vi "alignment by unt corner.vi"(8 "error in (no error)":errorcluster) -> (0 "error out":errorcluster, 3 "angle Z":ext, 5 "ant corner 2":ext, 11 "ant corner":ext)   [LabVIEW 2017]
uses:
  <vilib>/myRIO/Instrument Drivers/Onboard IO/I2C/typedefs/I2C Reference.ctl
  <vilib>/myRIO/Common/Instrument Driver Framework/Utilities/typedefs/myRIO Generic Hardware Reference.ctl
  <vilib>/myRIO/Common/Instrument Driver Framework/Utilities/typedefs/Hardware Version Enum.ctl
  <vilib>/myRIO/Common/Instrument Driver Framework/Utilities/typedefs/myRIO v1.0 Reference.ctl
  <vilib>/myRIO/Common/Instrument Driver Framework/Utilities/typedefs/Generic FPGA Reference.ctl
  <vilib>/myRIO/Common/Instrument Driver Framework/myRIO v1.0/I2C/typedefs/I2C Channels Enum.ctl
  <vilib>/myRIO/Instrument Drivers/Onboard IO/I2C/typedefs/I2C Configuration.ctl
  <vilib>/myRIO/Instrument Drivers/Onboard IO/I2C/typedefs/I2C Transfer Rate.ctl
  <vilib>/userdefined/High Color/nirio_resource_hc.ctl
  <vilib>/myRIO/Instrument Drivers/Onboard IO/DIO/typedefs/DIO Reference.ctl
  <vilib>/myRIO/Common/Instrument Driver Framework/myRIO v1.0/DIO/typedefs/DIO Channels List.ctl
  <vilib>/myRIO/Common/Instrument Driver Framework/myRIO v1.0/DIO/typedefs/DIO Channels Enum.ctl
  <vilib>/myRIO/Common/Instrument Driver Framework/myRIO v1.0/I2C/vis/myRIO v1.1 Open I2C.vi
  <vilib>/myRIO/Common/Instrument Driver Framework/Utilities/vis/Is FPGA Ref Available.vi
  <vilib>/myRIO/Common/Instrument Driver Framework/myRIO v1.0/DIO/vis/myRIO v1.1 Open DIO.vi
  <vilib>/myRIO/Instrument Drivers/Onboard IO/DIO/vis/Write.vi
  <vilib>/myRIO/Common/Instrument Driver Framework/Utilities/vis/Validate Channels.vi
  <vilib>/myRIO/Common/Instrument Driver Framework/myRIO v1.0/I2C/vis/myRIO v1.0 Reserve I2C.vi
  <vilib>/myRIO/Common/Instrument Driver Framework/myRIO v1.0/DIO/vis/myRIO v1.0 Reserve DIO.vi
  <vilib>/myRIO/Common/Instrument Driver Framework/myRIO v1.0/I2C/vis/myRIO v1.0 Close I2C.vi
  <vilib>/myRIO/Common/Instrument Driver Framework/myRIO v1.0/I2C/vis/myRIO v1.0 Build MUX Configuration I2C.vi
  <vilib>/myRIO/Common/Instrument Driver Framework/myRIO v1.0/Resource Manager/vis/myRIO v1.0 Reserve Channel List.vi
  <vilib>/myRIO/Common/Instrument Driver Framework/myRIO v1.0/DIO/vis/myRIO v1.0 Build MUX Configuration DIO.vi
  <vilib>/myRIO/Common/Instrument Driver Framework/myRIO v1.0/I2C/vis/myRIO v1.0 Unreserve I2C.vi
  <vilib>/myRIO/Common/Instrument Driver Framework/myRIO v1.0/Resource Manager/vis/myRIO v1.0 Create Configuration List.vi
  <vilib>/myRIO/Common/Instrument Driver Framework/myRIO v1.0/Resource Manager/vis/myRIO v1.0 Reserve Channel.vi
  <vilib>/myRIO/Common/Instrument Driver Framework/myRIO v1.0/Resource Manager/vis/myRIO v1.0 Unreserve Channel.vi
  <vilib>/myRIO/Common/Instrument Driver Framework/myRIO v1.0/Resource Manager/vis/myRIO v1.0 Unreserve Channel List.vi
  <vilib>/myRIO/Common/Instrument Driver Framework/myRIO v1.0/Resource Manager/vis/myRIO v1.0 Build Mutex Name.vi
  <vilib>/Utility/VariantDataType/GetNumericInfo.vi
  <vilib>/Utility/error.llb/Error Cluster From Error Code.vi
  <vilib>/myRIO/Common/Instrument Driver Framework/myRIO v1.0/myRIO v1.1 Open.vi
  <vilib>/myRIO/Common/Instrument Driver Framework/Utilities/vis/IO Manager.vi
  <vilib>/myRIO/Common/Instrument Driver Framework/Utilities/vis/Configuration Manager.vi
  <vilib>/myRIO/Common/Instrument Driver Framework/myRIO v1.0/Resource Manager/vis/myRIO v1.0 Configure IO.vi
  <vilib>/myRIO/Common/Instrument Driver Framework/myRIO v1.0/myRIO v1.0 Close.vi
  <vilib>/myRIO/Common/Instrument Driver Framework/myRIO v1.0/DIO/vis/myRIO v1.0 Write DIO.vi
  <vilib>/imath/engines/lvmath2/RunTimeEngine/Managers/WorkSpace/UID Generator.vi
  <vilib>/imath/engines/lvmath2/RunTimeEngine/RunTimeType/NIMS_RunTimeType_From StrictType (excl LVString).vi
  <instcachedir>/0/NIMS_RunTimeType_From StrictType (excl LVString)_1019F277F0A747EDBCA0F6C52CA54500.lvgen/NIMS_RunTimeType_From StrictType (excl LVString)_1019F277F0A747EDBCA0F6C52CA54500_000.vi
  <vilib>/imath/engines/lvmath2/RunTimeEngine/LocalVariableDefStatement/MC_LocalVariableDefStatement_Display.vi
  <vilib>/imath/engines/lvmath2/RunTimeEngine/RunTimeType/NIMS_RunTimeType_Set Source Original Bool.vi
  <vilib>/imath/engines/lvmath2/RunTimeEngine/Managers/SymbolTable/Clear UID.vi
  <vilib>/imath/engines/lvmath2/RunTimeEngine/NodeEndStatement/NIMS_NodeEndStatement_Output.vi
  <instcachedir>/0/NIMS_NodeEndStatement_Output_53EC0D466D134D7ABD903AC30B43404B.lvgen/NIMS_NodeEndStatement_Output_53EC0D466D134D7ABD903AC30B43404B_010.vi
  <vilib>/imath/engines/lvmath2/RunTimeEngine/ErrorHandling/NIMS_Finalize Error.vi
  <vilib>/myRIO/Common/Instrument Driver Framework/myRIO v1.0/I2C/vis/myRIO v1.0 Shutdown I2C.vi
  <vilib>/myRIO/Instrument Drivers/Onboard IO/I2C/vis/myRIO I2C Open.xnode
  <vilib>/myRIO/Express VI/Onboard Devices/LED/LED Express VI.xnode
  <vilib>/myRIO/Instrument Drivers/Onboard IO/DIO/vis/myRIO DIO Open.xnode
  <vilib>/myRIO/Instrument Drivers/Onboard IO/DIO/DIO.lvlib
  <vilib>/myRIO/Instrument Drivers/Onboard IO/I2C/I2C.lvlib
  <vilib>/imath/engines/lvmath2/RunTimeEngine/Managers/SymbolTable/NIMS_WorkSpace.lvlib
panel:
  in  "Stop Button":bool
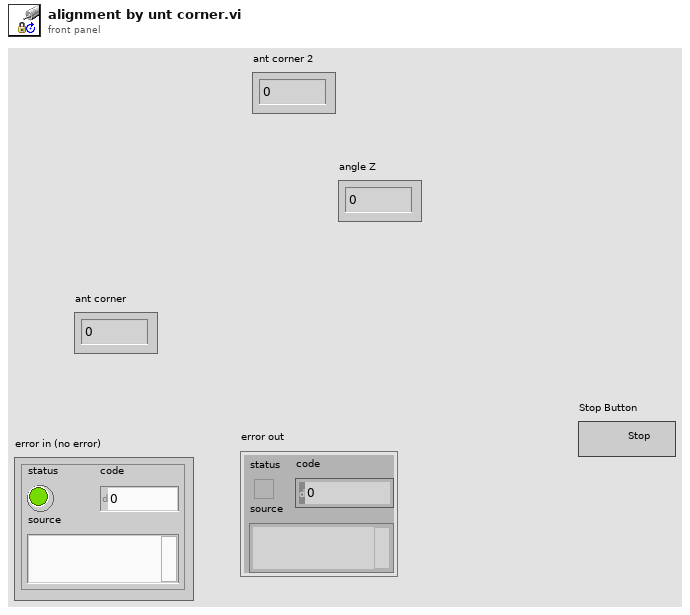
[diagram p1: front panel]
types:
  T1 = typedef "I2C.lvlib/I2C Reference.ctl" = cluster{"myRIO Reference":T2, "I2C Channels Enum":T6, "I2C Configuration":T7}
  T2 = typedef "myRIO Generic Hardware Reference.ctl" = cluster{"myRIO Model":T3, "myRIO Hardware Reference":T4}
  T3 = typedef "Hardware Version Enum.ctl" = enum16{"Unknown", "myRIO-1900", "myRIO-1950", "roboRIO", "NI ELVIS RIO CM"}
  T4 = typedef "myRIO v1.0 Reference.ctl" = cluster{"Generic FPGA Reference":T5, "Allow multiple opens":bool}
  T5 = typedef "Generic FPGA Reference.ctl" = refnum<k20>
  T6 = typedef "I2C Channels Enum.ctl" = enum16{"Not Connected", "A/I2C", "B/I2C", "I2C/I2C"}
  T7 = typedef "I2C.lvlib/I2C Configuration.ctl" = cluster{"I2C Transfer Rate":T8}
  T8 = typedef "I2C.lvlib/I2C Transfer Rate.ctl" = enum16{"Standard mode (100 kbps)", "Fast mode (400 kbps)"}
  T9 = typedef "DIO.lvlib/DIO Reference.ctl" = cluster{"myRIO Reference":T2, "DIO Channels List":T10}
  T10 = typedef "DIO Channels List.ctl" = T11[]
  T11 = typedef "DIO Channels Enum.ctl" = enum16{"Not Connected", "C/DIO0", "C/DIO1", "C/DIO2", "C/DIO3", "C/DIO4", "C/DIO5", "C/DIO6", "C/DIO7", "A/DIO0", "A/DIO1", "A/DIO2", "A/DIO3", "A/DIO4", "A/DIO5", "A/DIO6", "A/DIO7", "A/DIO8", "A/DIO9", "A/DIO10", "A/DIO11", "A/DIO12", "A/DIO13", "A/DIO14", "A/DIO15", "B/DIO0", "B/DIO1", "B/DIO2", "B/DIO3", "B/DIO4", "B/DIO5", "B/DIO6", "B/DIO7", "B/DIO8", "B/DIO9", "B/DIO10", "B/DIO11", "B/DIO12", "B/DIO13", "B/DIO14", "B/DIO15", "LED0", "LED1", "LED2", "LED3", "Button0", "DIO/DIO0", "DIO/DIO1", "DIO/DIO2", "DIO/DIO3", "DIO/DIO4", "DIO/DIO5", "DIO/DIO6", "DIO/DIO7", "DIO/DIO8", "DIO/DIO9", "SPI/CS0", "SPI/CS1", "SPI/CS2", "SPI/CS3", "LED RADIO (Green)", "LED RADIO (Red)", "LED COMM (Green)", "LED COMM (Red)", "LED MODE (Green)", "LED MODE (Red)"}
  T12 = typedef "nirio_resource_hc.ctl" = tag
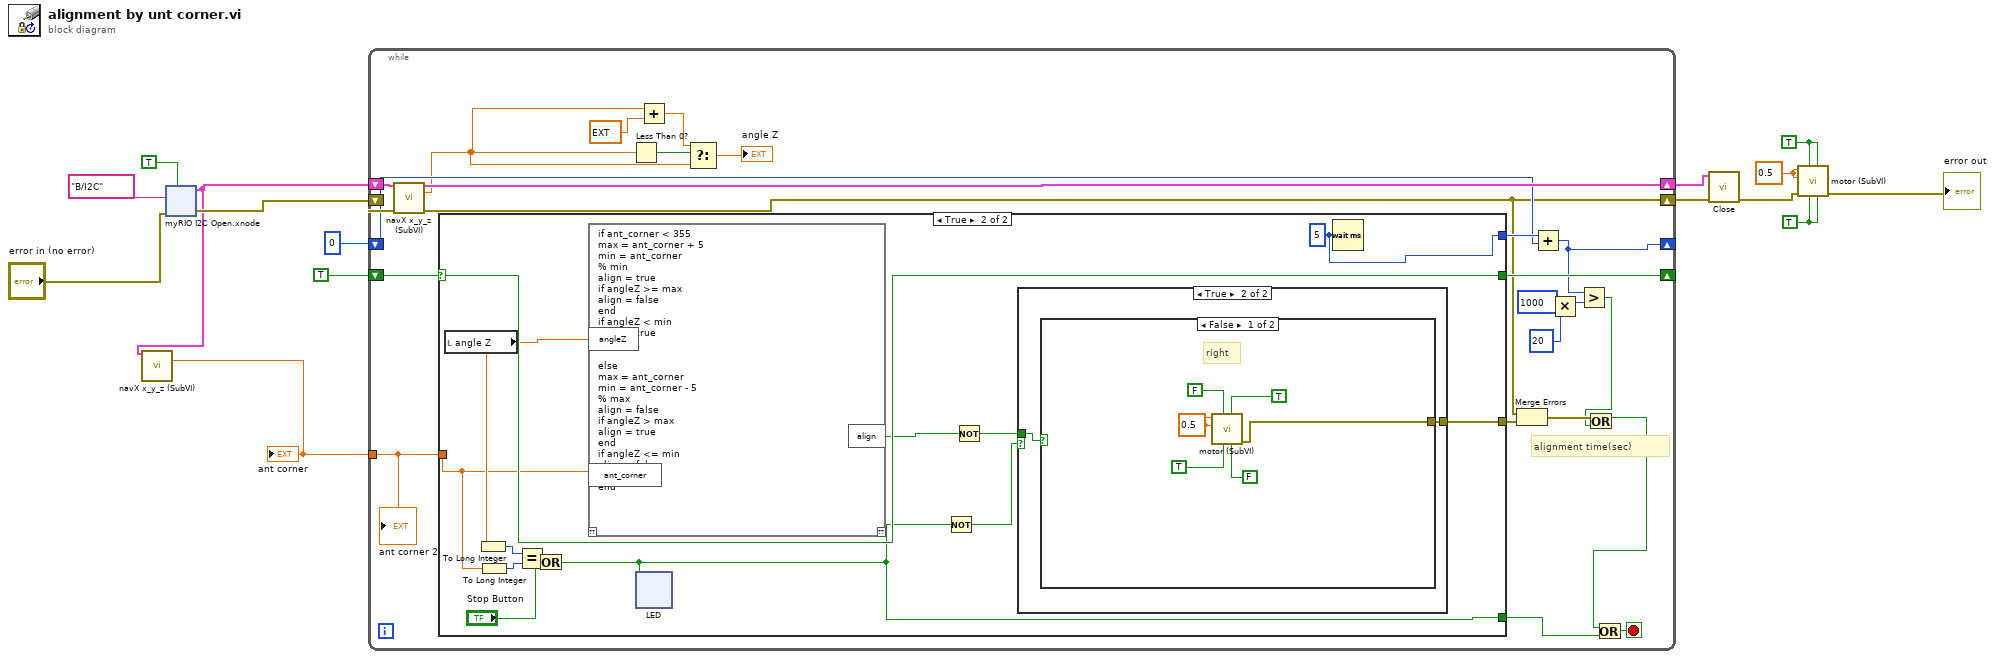
[diagram p0: block diagram]
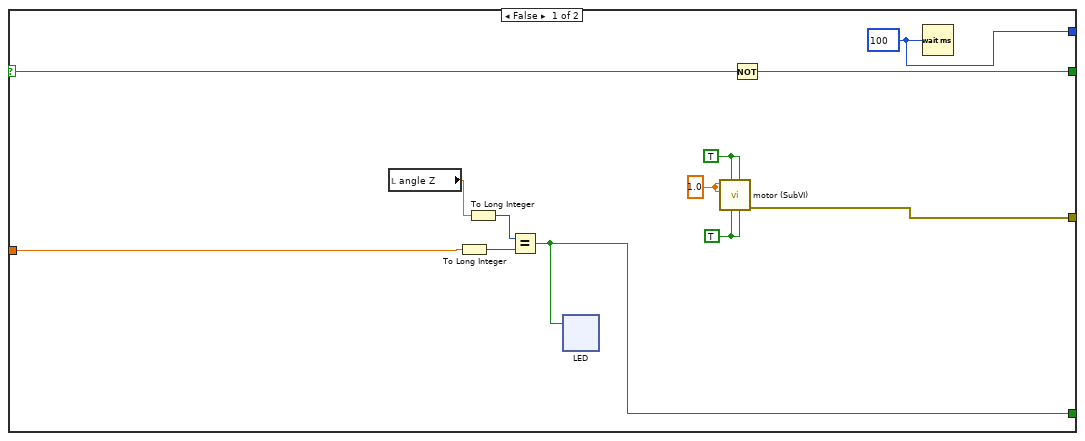
[diagram p2: hidden frame]
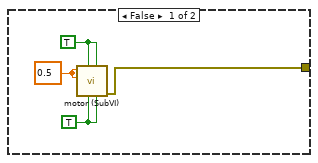
[diagram p3: hidden frame]
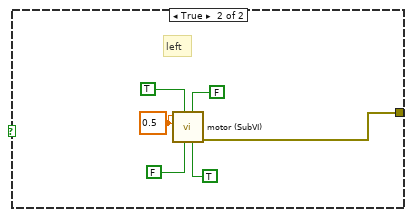
[diagram p4: hidden frame]
diagram:
  w5 = 0.5 ("PWM0")
  w6 = TRUE ("M0 (Pin 23)")
  w7 = TRUE ("M1 (Pin 25)")
  n1 = xnode "myRIO I2C Open.xnode"("error in (no error)"="error in (no error)", "Allow multiple opens?"=TRUE, "Channel Name"=tag "B/I2C") -> ("error out"=w12:errorcluster, "I2C Ref Out"=w2:T1)
  n2 = call "navX x_y_z (SubVI).vi"("I2C Ref Out in"=w2) -> ("value Z"=w1:ext)  [unwired: 10 in, 4 out]
  "ant corner" <- w1
  n3 = while {
    shift-right: [w37] -> _
    shift-left: TRUE -> [w38]
    tunnel: w1 -> [w36]
    shift-right: [w24] -> _
    shift-left: u32 0 ("y") -> [w25]
    shift-right: [w35] -> w8
    shift-left: w2 -> [w18]
    shift-right: [w17] -> w15
    shift-left: w12 -> [w39]
    stop <- w34 stop-if-true
    # "alignment time(sec)"
    n4 = call "navX x_y_z (SubVI).vi"("I2C Ref Out in"=w18, "error in (no error)"=w39) -> ("I2C Ref Out out"=w35:T1, "value Z"=w16:ext, "error out"=w17:errorcluster)  [unwired: 9 in, 2 out]
    n5 = case shown="True" w38 {
      selector: w38 -> [w47 w99]
      tunnel: [w51 w98] -> w31
      tunnel: [w46 w99] -> w37
      tunnel: w36 -> [w43 w89]
      tunnel: [w40 w92] -> w32
      tunnel: [w45 w93] -> w26
      frame False {
        w45 = u32 100 ("milliseconds to wait")
        w48 = 1.0 ("PWM0")
        w49 = TRUE ("M0 (Pin 23)")
        w50 = TRUE ("M1 (Pin 25)")
        n6 = local read "angle Z"() -> (w44:ext)
        n7 = To Long Integer(number=w43) -> (32bit integer=w41:i32)
        n8 = To Long Integer(number=w44) -> (32bit integer=w42:i32)
        n9 = Equal?(x=w42, y=w41) -> (x = y?=w40:bool)
        n10 = xnode "LED"("LED3"=w40) -> ()  [unwired: 1 in, 1 out]
        n11 = call "motor (SubVI).vi"("M1 (Pin 26)"=w49, "M1 (Pin 25)"=w50, "M0 (Pin 23)"=w49, "M0 (Pin 21)"=w50, "PWM1"=w48, "PWM0"=w48) -> ("error out"=w51:errorcluster)  [unwired: 5 in]
        n12 = Not(x=w47) -> (.not. x?=w46:bool)
        n13 = Wait (ms)(milliseconds to wait=w45) -> ()  [unwired: 1 out]
      }
      frame True {
        w93 = u32 5 ("milliseconds to wait")
        n14 = local read "angle Z"() -> (w90:ext)
        n15 = To Long Integer(number=w90) -> (32bit integer=w97:i32)
        n16 = To Long Integer(number=w89) -> (32bit integer=w96:i32)
        n17 = Equal?(x=w97, y=w96) -> (x = y?=w95:bool)
        n18 = Or(x=w95, y="Stop Button") -> (x .or. y?=w92:bool)
        n19 = mathscript code="if ant_corner < 355\nmax = ant_corner + 5\nmin = ant_corner\n% min\nalign = true\nif angleZ >= max\nalign = false\nend\nif angleZ < min\nalign = true\nend\n\nelse\nmax = ant_corner\nmin = ant_corner - 5\n% max\nalign = false\nif angleZ > max\nalign = true\nend\nif angleZ <= min\nalign = false\nend\nend"("angleZ"=w90, "ant_corner"=w89) -> ("align"=w88:bool)  [unwired: 1 in, 1 out]
        n20 = xnode "LED"("LED3"=w92) -> ()  [unwired: 1 in, 1 out]
        n21 = Not(x=w92) -> (.not. x?=w91:bool)
        n22 = Not(x=w88) -> (.not. x?=w87:bool)
        n23 = case shown="True" w91 {
          tunnel: w87 -> [_ w384]
          tunnel: [w379 w383] -> w98
          frame False {
            w380 = 0.5 ("PWM0")
            w381 = TRUE ("M0 (Pin 23)")
            w382 = TRUE ("M1 (Pin 25)")
            n24 = call "motor (SubVI).vi"("M1 (Pin 26)"=w381, "M1 (Pin 25)"=w382, "M0 (Pin 23)"=w381, "M0 (Pin 21)"=w382, "PWM1"=w380, "PWM0"=w380) -> ("error out"=w379:errorcluster)  [unwired: 5 in]
          }
          frame True {
            n25 = case shown="False" w384 {
              tunnel: [w385 w396] -> w383
              frame False {
                w386 = 0.5 ("PWM1")
                # "right"
                n26 = call "motor (SubVI).vi"("M1 (Pin 26)"=FALSE ("M1 (Pin 25)"), "M1 (Pin 25)"=TRUE ("right"), "M0 (Pin 23)"=TRUE ("right"), "M0 (Pin 21)"=FALSE, "PWM1"=w386, "PWM0"=w386) -> ("error out"=w385:errorcluster)  [unwired: 5 in]
              }
              frame True {
                w391 = 0.5 ("PWM1")
                # "left"
                n27 = call "motor (SubVI).vi"("M1 (Pin 26)"=TRUE ("M1 (Pin 25)"), "M1 (Pin 25)"=FALSE, "M0 (Pin 23)"=FALSE ("M1 (Pin 25)"), "M0 (Pin 21)"=TRUE ("M1 (Pin 25)"), "PWM1"=w391, "PWM0"=w391) -> ("error out"=w396:errorcluster)  [unwired: 5 in]
              }
            }
          }
        }
        n28 = Wait (ms)(milliseconds to wait=w93) -> ()  [unwired: 1 out]
      }
    }
    n29 = Less Than 0?(x=w16) -> (x < 0?=w30:bool)
    n30 = Add(x=w16, y=ext 360.0) -> (x+y=w29:ext)
    n31 = Select(t=w29, s=w30, f=w16) -> (s? t:f=→"angle Z":ext)
    n32 = Merge Errors(w17, w31) -> (w33:errorcluster)
    n33 = Add(x=w26, y=w25) -> (x+y=w24:u32)
    n34 = Multiply(x=u32 1000, y=u32 20) -> (x*y=w22:u32)
    n35 = Greater?(x=w24, y=w22) -> (0:w19:bool)
    n36 = Or(x=w33, y=w19) -> (x .or. y?=w20:bool)
    n37 = Or(x=w20, y=w32) -> (x .or. y?=w34:bool)
    "ant corner 2" <- w36
  }
  n38 = call <vilib>:"Close.vi"("error in (no error)"=w15, "I2C Ref In"=w8) -> ("error out"=w3:errorcluster)  [unwired: 9 in]
  n39 = call "motor (SubVI).vi"("M1 (Pin 26)"=w6, "M1 (Pin 25)"=w7, "M0 (Pin 23)"=w6, "M0 (Pin 21)"=w7, "error in (no error)"=w3, "PWM1"=w5, "PWM0"=w5) -> ("error out"=→"error out":errorcluster)  [unwired: 4 in]
